vi "flow-gen.nutrition-dosing.vi"(9 "Unit Index":i32, 10 "Dosing Time":dbl, 11 "IO Name":string) -> (2 "Should Dose?":bool, 3 "Flow":T1[](array[typedef]))   [LabVIEW 2024]
uses:
  controls/UiStepBuilder.ctl
  controls/type.step-builder.ctl
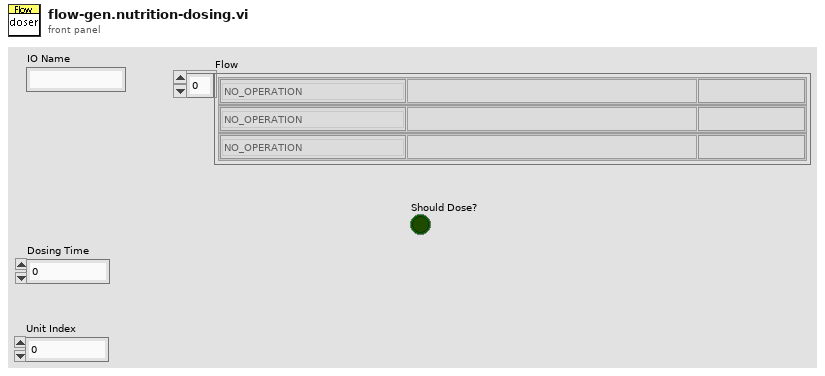
[diagram p1: front panel]
types:
  T1 = typedef "UiStepBuilder.ctl" = cluster{"Step Function":T2, "ParamString":string, "Step Label":string}
  T2 = typedef "type.step-builder.ctl" = enum16{"NO_OPERATION", "DELAY-JUMP", "DELAY", "JUMP", "COMPLETE", "SCHEDULER", "IRR-CHECK", "UNIT-CHECK", "UNIT-SAMPLE", "UNIT-DOSE", "LOG-REPORT", "LOG-MESSAGE", "IO-READ", "IO-READ-MANY", "IO-WRITE", "IO-COMPARE-OUT", "IO-COMPARE-IN", "PROC-START", "PROC-STOP", "PROC-LOAD", "PROC-IS-COMPLETED", "RECORD-MOVE", "GET-RH", "GET-UV", "GET-WD", "GET-WS", "OCS-CHECK", "OCS-RECORD"}
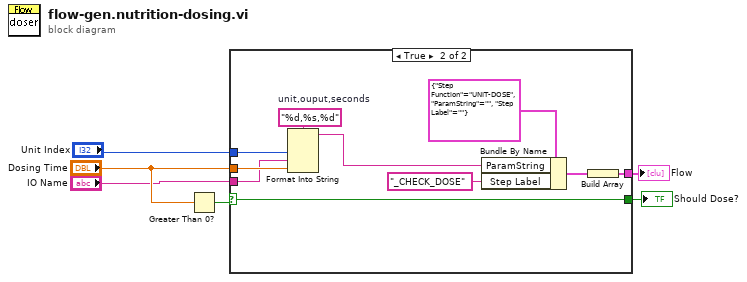
[diagram p0: block diagram]
diagram:
  n1 = Greater Than 0?(x="Dosing Time") -> (x > 0?=w4:bool)
  n2 = case shown="True" w4 {
    selector: w4 -> [_ w8]
    tunnel: "Dosing Time" -> [_ w11]
    tunnel: [_ w13] -> w3
    tunnel: "IO Name" -> [_ w10]
    tunnel: "Unit Index" -> [_ w9]
    tunnel: [_ w8] -> w1
    frame False {
    }
    frame True {
      w15 = "%d,%s,%d"  # unit,ouput,seconds
      n3 = Format Into String(format string=w15, w9, w10, w11) -> (resulting string=w12:string)  [unwired: 2 in, 1 out]
      n4 = Bundle By Name(cluster=T1 {"Step Function"=enum."UNIT-DOSE", "ParamString"="", "Step Label"=""} ("FlowModeConstant 2"), "ParamString"=w12, "Step Label"="_CHECK_DOSE") -> (w14:T1)
      n5 = Build Array(w14) -> (w13:T1[])
    }
  }
  "Flow" <- w3
  "Should Dose?" <- w1
